vi "newDangerEnemy.vi"(0 "MarkerSkill in":refnum<class "MarkerSkill.lvclass">, 5 "Game":refnum<class "Game.lvclass">, 11 "error in (no error)":errorcluster) -> (4 "MarkerSkill out":refnum<class "MarkerSkill.lvclass">, 6 "dangerEnemies":T1[](array[typedef]), 8 "numberOfPossible\nEnemiesToMark":i32, 15 "error out":errorcluster)   [LabVIEW 2020, in "MarkerSkill.lvclass"]
uses:
  MarkerSkill.lvclass
  Ally_class/Ally.lvclass
  Game_class/Game.lvclass
  Enemy_class/Enemy.lvclass
  dangerEnemy.ctl
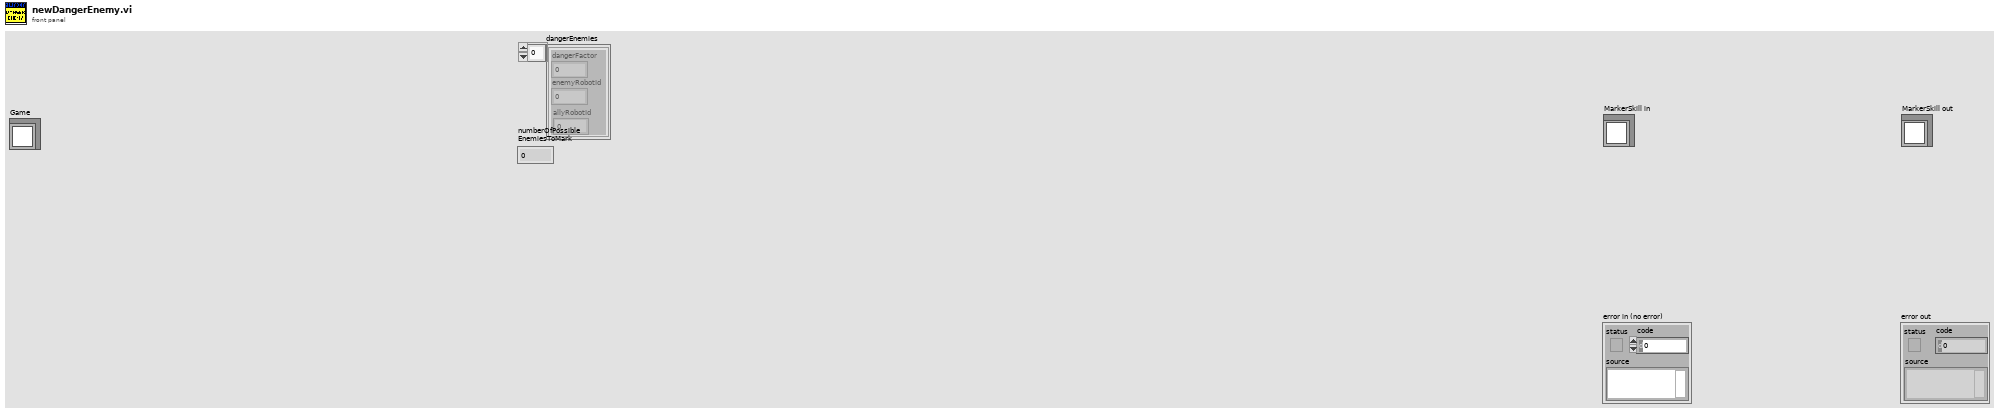
[diagram p1: front panel]
types:
  T1 = typedef "dangerEnemy.ctl" = cluster{"dangerFactor":dbl, "allyRobotId":i32, "enemyRobotId":i32}
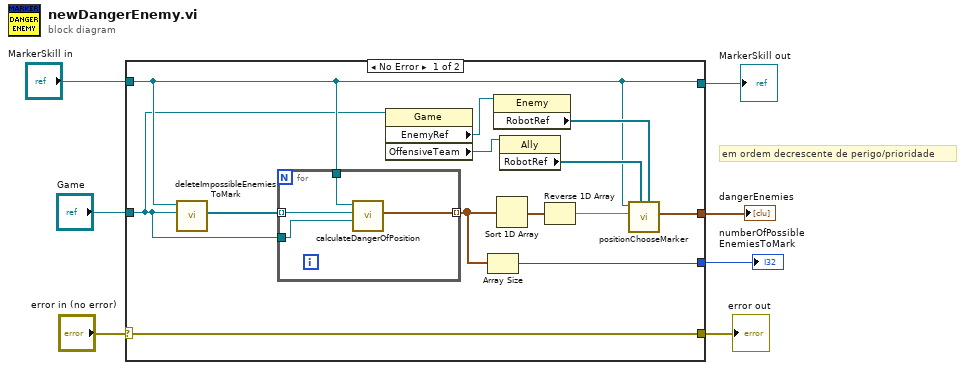
[diagram p0: block diagram]
diagram:
  # "em ordem decrescente de perigo/prioridade"
  n1 = case shown="No Error" "error in (no error)" {
    selector: "error in (no error)" -> [w20 w26]
    tunnel: [w20 w26] -> w6
    tunnel: [w9 w25] -> w4
    tunnel: "MarkerSkill in" -> [w9 w25]
    tunnel: "Game" -> [w8 _]
    tunnel: [w14 _] -> w2
    tunnel: [w16 _] -> w1
    frame No Error {
      n2 = call "deleteImpossibleEnemiesToMark.vi"("Game"=w8, "MarkerSkill in"=w9) -> ("PossibleEnemiesToMark"=w18:refnum<class "Robot.lvclass">[])  [unwired: 7 in, 2 out]
      n3 = for {
        tunnel: w9 -> [w24]
        tunnel: [w23] -> w17 mode=indexing
        tunnel: w18 -> [w22] mode=indexing
        tunnel: w8 -> [w21]
        n4 = call "calculateDangerOfPosition.vi"("Game"=w21, "Enemy Robot"=w22, "MarkerSkill in"=w24) -> ("DangerEnemy"=w23:T1)  [unwired: 6 in, 2 out]
      }
      n5 = property class="Game"(reference=w8) -> ("EnemyRef"=w11:refnum<class "Enemy.lvclass">, "OffensiveTeam"=w13:refnum<class "Ally.lvclass">)  [unwired: 1 in, 2 out]
      n6 = Array Size(array=w17) -> (size(s)=w16:i32)
      n7 = property class="Enemy"(reference=w11) -> ("RobotRef"=w10:refnum<class "Robot.lvclass">[])  [unwired: 1 in, 2 out]
      n8 = Sort 1D Array(array=w17) -> (sorted array=w19:T1[])
      n9 = property class="Ally"(reference=w13) -> ("RobotRef"=w12:refnum<class "Robot.lvclass">[])  [unwired: 1 in, 2 out]
      n10 = Reverse 1D Array(array=w19) -> (reversed array=w15:T1[])
      n11 = call "positionChooseMarker.vi"("enemyRobots"=w10, "OffensiveRobots"=w12, "dangerEnemies in"=w15, "MarkerSkill in"=w9) -> ("dangerEnemies out"=w14:T1[])  [unwired: 5 in, 2 out]
    }
    frame Error {
    }
  }
  "error out" <- w6
  "MarkerSkill out" <- w4
  "dangerEnemies" <- w2
  "numberOfPossible\nEnemiesToMark" <- w1
